vi "stop rec.vi"(11 "hwnd":u32) -> (3 "hwnd 2":u32)   [LabVIEW 2011]
uses:
  user32.dll
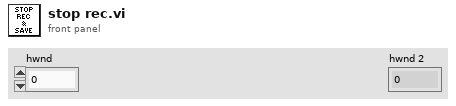
[diagram p1: front panel]
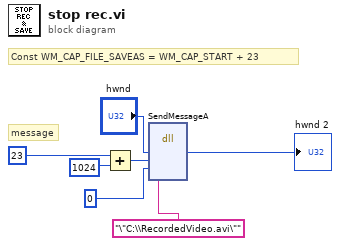
[diagram p0: block diagram]
diagram:
  # "message"
  # "Const WM_CAP_FILE_SAVEAS = WM_CAP_START + 23"
  n1 = Add(x=u32 23, y=u32 1024 ("msg")) -> (x+y=w4:u32)
  n2 = dll-call lib="user32.dll" fn="SendMessageA"("hwnd"="hwnd", "msg"=w4, "wParam"=u32 0, "lparam"="\"C:\\RecordedVideo.avi\"") -> ("hwnd"=→"hwnd 2":u32)  [unwired: 7 in, 2 out]
